vi "beads_DAQ.vi"() -> ()   [LabVIEW 2014]
panel:
  in  "Flash lamp\n settings:":T1={"Flash lamp?"=FALSE, "Number of cyles\nbetween flashes"=3, "# Pulses"=3, "Stop flashing \nbelow thresh?"=FALSE, "Stop threshold"=0.05}
  in  "Stage settings:":T2={"Set stage?"=FALSE, "start X (um)"=0.0, "stop X (um) "=0.0, "# X Steps"=1, "start Y (um)"=0.0, "stop Y (um) "=0.0, "# Y steps"=1, "start Z (um)"=0.0, "stop Z (um)"=0.0, "# Z steps "=1}
  in  "Electrode settings:":T3={"DC volts (V):\n"=[[0.0, 0.0, 0.0, 0.0, 0.0, 0.0, 0.0, 0.0], [0.0, 0.0, 0.0, 0.0, 0.0, 0.0, 0.0, 0.0]], "Sweep electrode? "=FALSE, "Electrode to sweep:"=0, "start volt (V)"=0.0, "stop volt (V) "=0.0, "# V Steps"=1, "start freq (Hz)"=41.0, "stop freq (Hz) "=41.0, "# F steps"=1, "start DC (V)"=0.0, "stop DC (V)"=0.0, "# DC steps "=1}
  in  "DC supply settings:":T4
  in  "Synth settings:":T5={"start volt (V)"=0.0, "stop volt (V) "=0.0, "# V Steps"=1, "start freq (Hz)"=41.0, "stop freq (Hz) "=41.0, "# F steps"=1, "dc offset?"=FALSE, "start DC (V)"=0.0, "stop DC (V)"=0.0, "# DC steps "=1, "Set synth\n(HP33120A)?"=FALSE}
  out "Waveform Graph":dbl[][](graph)
  out "Curr threshold":dbl
  in  "Number of Samples":i32=50000
  in  "Sample Rate [Hz]":dbl=5000.0
  out "Actual Sample Rate":dbl=5000.0 format="%0.2f"
  in  "Delay time between files [s]":dbl caption="Delay Time (s)"
  in  "Num files":i32=1
  in  "File base name":string="junk"
  in  "Directory path":path=path "C:/Data/test"
  # "Flash Lamp Settings"
  # "0"
  # "1"
  # "2"
  # "3"
  # "4"
  # "5"
  # "6"
  # "7"
  # "Acquired Data"
  # "Timing Settings"
  # "Logging Settings"
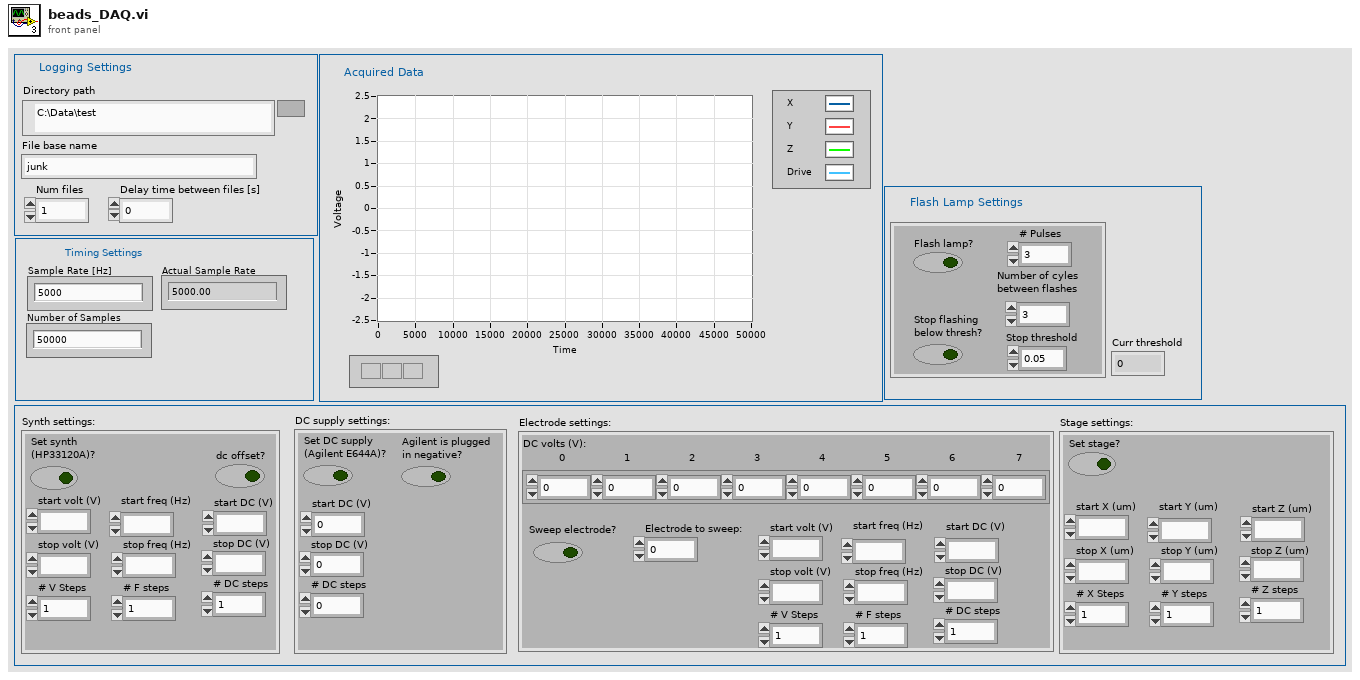
[diagram p1: front panel]
types:
  T1 = cluster{"Flash lamp?":bool, "Number of cyles\nbetween flashes":i32, "# Pulses":i32, "Stop flashing \nbelow thresh?":bool, "Stop threshold":dbl}
  T2 = cluster{"Set stage?":bool, "start X (um)":ext, "stop X (um) ":ext, "# X Steps":i32, "start Y (um)":ext, "stop Y (um) ":ext, "# Y steps":i32, "start Z (um)":ext, "stop Z (um)":ext, "# Z steps ":i32}
  T3 = cluster{"DC volts (V):\n":dbl[][], "Sweep electrode? ":bool, "Electrode to sweep:":i32, "start volt (V)":ext, "stop volt (V) ":ext, "# V Steps":i32, "start freq (Hz)":ext, "stop freq (Hz) ":ext, "# F steps":i32, "start DC (V)":ext, "stop DC (V)":ext, "# DC steps ":i32}
  T4 = cluster{"start DC (V)":ext, "stop DC (V)":ext, "# DC steps ":i32, "Set DC supply\n(Agilent E644A)? ":bool, "Agilent is plugged \nin negative?":bool}
  T5 = cluster{"start volt (V)":ext, "stop volt (V) ":ext, "# V Steps":i32, "start freq (Hz)":ext, "stop freq (Hz) ":ext, "# F steps":i32, "dc offset?":bool, "start DC (V)":ext, "stop DC (V)":ext, "# DC steps ":i32, "Set synth\n(HP33120A)?":bool}
  T6 = cluster{"Tot Synth Arr":dbl[], "Tot DC Arr":dbl[], "Tot Electrode Arr":dbl[], "Tot Stage Arr":dbl[]}[]
  T7 = cluster{"dup VISA session":refnum<visa-resource-name>, "error out":errorcluster, "task out":refnum<k21>, "error out":errorcluster}
  T8 = cluster{"Number of Samples":i32, "Sample Rate [Hz]":dbl, "Physical Channels (Position signals)":tag, "Physical Channel (drive signals)":tag, "Sample Clock Source":tag, "Physical Channel (drive signals)":tag}
  T9 = cluster{"Flash lamp\n settings:":cluster{"Flash lamp?":bool, "Number of cyles\nbetween flashes":i32, "# Pulses":i32, "Stop flashing \nbelow thresh?":bool, "Stop threshold":dbl}, "Output channel (for flashing)":tag, i32, "path out":path}
  T10 = cluster{"dup VISA session":refnum<visa-resource-name>, "error out":errorcluster, "Agilent is \nplugged in \nnegative?":bool, "electrodes task":refnum<k21>, "electrodes task error":errorcluster, "Set synth":bool, "Set DC":bool}
  T11 = cluster{"data task":refnum<k21>, "data task error":errorcluster, "drive task":refnum<k21>, "drive task error":errorcluster, "trigger task":refnum<k21>, "trigger task error":errorcluster, "sample rate":dbl}
  T12 = cluster{"task out":refnum<k21>, "error out":errorcluster, "task out":refnum<k21>, "error out":errorcluster, "trigger task":refnum<k21>, "trigger task error":errorcluster}
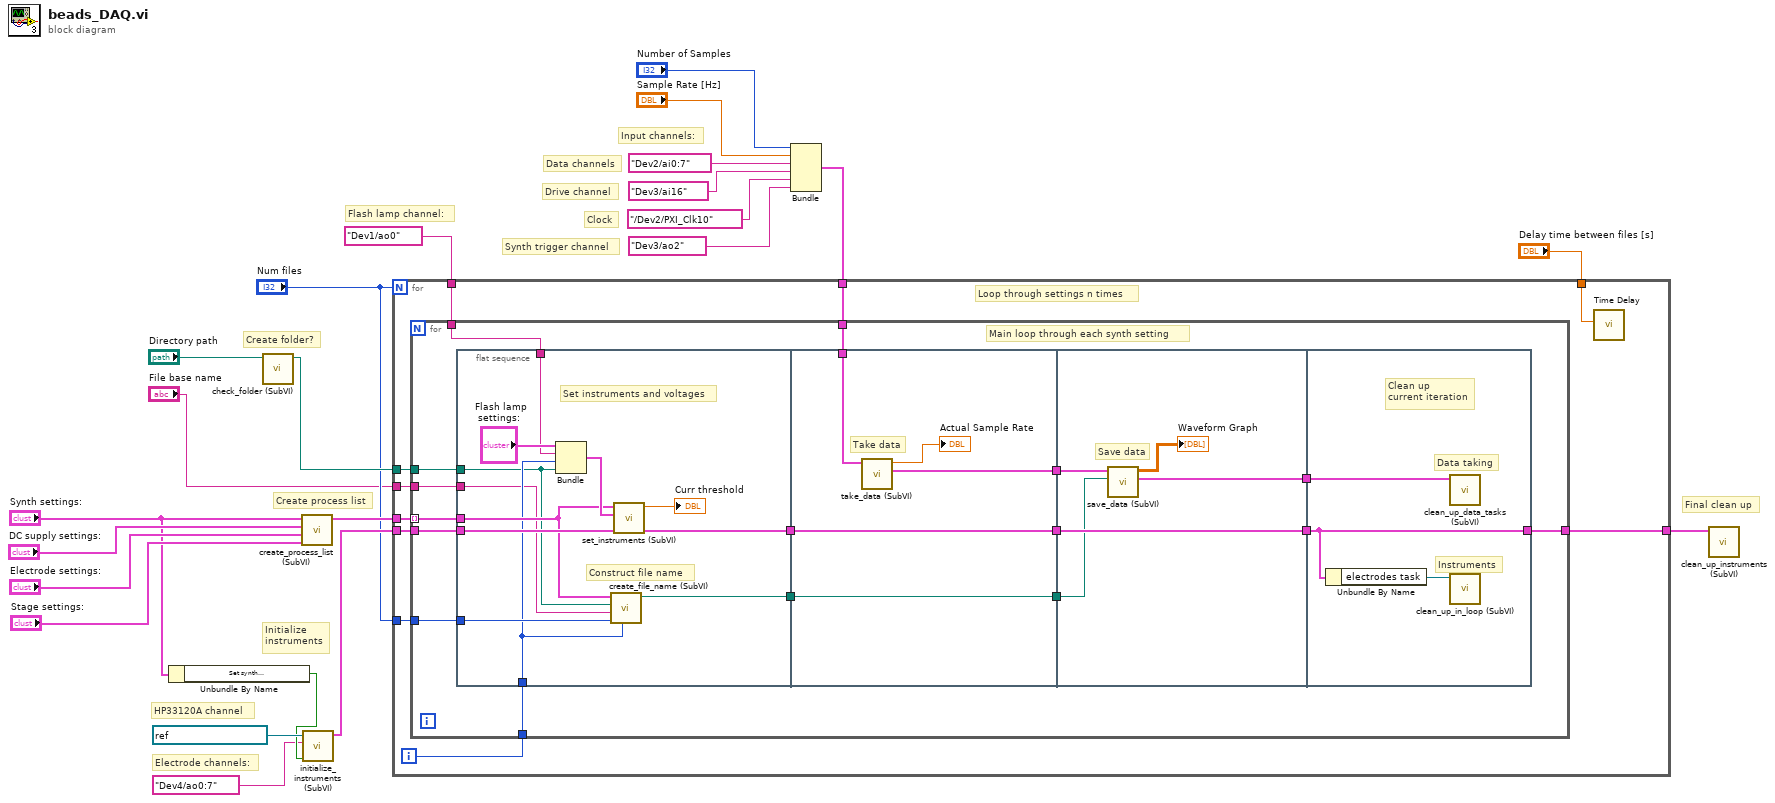
[diagram p0: block diagram]
diagram:
  # "Clock"
  # "Drive channel"
  # "Synth trigger channel"
  # "Data channels"
  # "Initialize\ninstruments"
  # "Electrode channels:"
  # "HP33120A channel"
  # "Flash lamp channel:"
  # "Create process list"
  # "Final clean up"
  # "Input channels:"
  # "Create folder?"
  n1 = Unbundle By Name("Synth settings:") -> ("Set synth\n(HP33120A)?"=w13:bool)
  n2 = call "check_folder (SubVI).vi"("path in"="Directory path") -> ("path out"=w16:path)  [unwired: 10 in]
  n3 = call "create_process_list (SubVI).vi"("Synth settings:"="Synth settings:", "DC supply settings:"="DC supply settings:", "Electrode settings:"="Electrode settings:", "Stage settings:"="Stage settings:") -> ("Process list"=w18:T6)  [unwired: 5 in]
  n4 = call "initialize_instruments (SubVI).vi"("Use synth?"=w13, "Electrode outupt channels"=tag "Dev4/ao0:7" ("Output channel (for flashing)"), "VISA Refnum in"=refnum<visa-resource-name> "GPIB0::10::INSTR" ("VISA session")) -> ("instrument config"=w12:T7)  [unwired: 8 in]
  n5 = Bundle("Number of Samples"="Number of Samples", "Sample Rate [Hz]"="Sample Rate [Hz]", "Physical Channels (Position signals)"=tag "Dev2/ai0:7", "Physical Channel (drive signals)"=tag "Dev3/ai16", "Sample Clock Source"=tag "/Dev2/PXI_Clk10", "Physical Channel (drive signals)"=tag "Dev3/ao2") -> (w4:T8)  [unwired: 1 in]
  n6 = for {
    N: "Num files" -> [_]
    tunnel: "Delay time between files [s]" -> [w33]
    tunnel: w18 -> [w32]
    tunnel: tag "Dev1/ao0" ("Output channel (for flashing)") -> [w31]
    tunnel: w16 -> [w29]
    tunnel: w12 -> [w28]
    tunnel: "Num files" -> [w27]
    tunnel: "File base name" -> [w26]
    tunnel: w4 -> [w25]
    tunnel: [w24] -> w1
    i -> [w30]
    # "Loop through settings n times"
    n7 = for {
      tunnel: w32 -> [w49] mode=indexing
      tunnel: w31 -> [w48]
      tunnel: w30 -> [w47]
      tunnel: w29 -> [w46]
      tunnel: w28 -> [w45]
      tunnel: w27 -> [w41]
      tunnel: w26 -> [w40]
      tunnel: w25 -> [w39]
      tunnel: [w34] -> w24
      # "Main loop through each synth setting"
      n8 = flat-sequence {
        tunnel: w49 -> [w55]
        tunnel: w48 -> [w60]
        tunnel: w47 -> [w53]
        tunnel: w46 -> [w52]
        tunnel: w45 -> [w57]
        tunnel: [w56] -> w42
        tunnel: w41 -> [w54]
        tunnel: w40 -> [w51]
        tunnel: [w50] -> w36
        tunnel: [w66] -> w43
        tunnel: w42 -> [w66]
        tunnel: w39 -> [w64]
        tunnel: [w63] -> w38
        tunnel: [w62] -> w37
        tunnel: w36 -> [w62]
        tunnel: [w71] -> w44
        tunnel: w43 -> [w71]
        tunnel: w38 -> [w70]
        tunnel: w37 -> [w68]
        tunnel: [w67] -> w35
        tunnel: w44 -> [w72]
        tunnel: w35 -> [w73]
        tunnel: [w72] -> w34
        frame #0 {
          # "Set instruments and voltages"
          # "Construct file name"
          n9 = Bundle("Flash lamp\n settings:"="Flash lamp\n settings:", "Output channel (for flashing)"=w60, w53, "path out"=w52) -> (w59:T9)  [unwired: 1 in]
          n10 = call "create_file_name (SubVI).vi"("file_idx"=w53, "num files"=w54, "base name"=w51, "Path"=w52, "Cluster"=w55) -> ("out path"=w50:path)  [unwired: 6 in]
          n11 = call "set_instruments (SubVI).vi"("instrument config"=w57, "Flash lamp settings:"=w59, "Process list"=w55) -> ("instrum out"=w56:T10, "Curr threshold"=→"Curr threshold":dbl)  [unwired: 7 in]
        }
        frame #1 {
          # "Take data"
          n12 = call "take_data (SubVI).vi"("channel settings"=w64) -> ("data tasks"=w63:T11, "Actual Sample Rate"=→"Actual Sample Rate":dbl)  [unwired: 9 in]
        }
        frame #2 {
          # "Save data"
          n13 = call "save_data (SubVI).vi"("Filename"=w68, "data tasks"=w70) -> ("output data tasks"=w67:T12, "Output data"=→"Waveform Graph":dbl[][])  [unwired: 8 in]
        }
        frame #3 {
          # "Instruments"
          # "Data taking"
          # "Clean up\ncurrent iteration"
          n14 = Unbundle By Name(w72) -> ("electrodes task"=w74:refnum<k21>)
          n15 = call "clean_up_data_tasks (SubVI).vi"("data tasks"=w73) -> ()  [unwired: 11 in]
          n16 = call "clean_up_in_loop (SubVI).vi"("Refnum in"=w74) -> ()  [unwired: 10 in, 1 out]
        }
      }
    }
    n17 = call "Time Delay"("Delay Time (s)"=w33) -> ()  [unwired: 10 in, 1 out]
  }
  n18 = call "clean_up_instruments (SubVI).vi"("instrum out"=w1) -> ()  [unwired: 11 in]
